vi "save config.vi"(8 "error in (no error)":errorcluster, 10 "file config":string, 11 "Channel in":refnum<class "Channel.lvclass">) -> (0 "error out":errorcluster, 3 "Channel out":refnum<class "Channel.lvclass">)   [LabVIEW 2018, in "Channel.lvclass"]
uses:
  Channel.lvclass
  Channel.lvclass/Channel.ctl
  <vilib>/Utility/config.llb/Write Key (String).vi
  Interface/Interface.lvclass
  <vilib>/Utility/config.llb/NI_LVConfig.lvlib
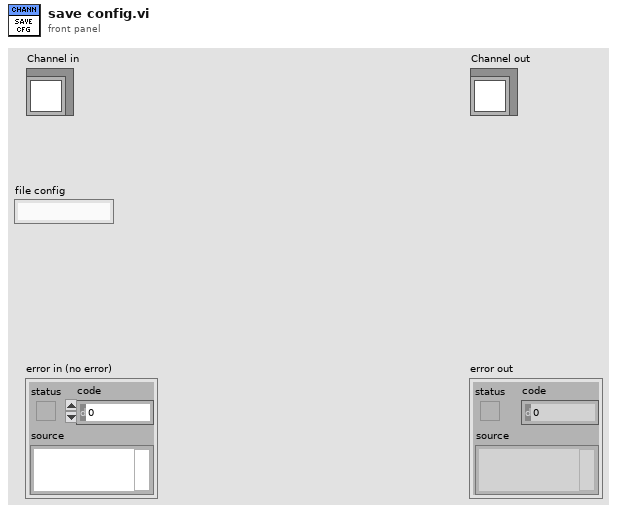
[diagram p1: front panel]
types:
  T1 = cluster{"ACQUISITION_MODE":u8, "TRIGGER_MODE":u8, "READ_MODE":u8, "PREAMP":u8, "READOUT_RATE":u8, "VERTICAL_SHIFT_SPEED":u8, "EM_MODE":u8, "EM_GAIN":u16, "SHUTTER_MODE":u8, "SHUTTER_TTL":u8, "SHUTTER_OPENNING_TIME":u16, "SHUTTER_CLOSING_TIME":u16, "VBIN":u16, "HBIN":u16, "INITIAL_LINE":u16, "INITIAL_COLUMN":u16, "FINAL_LINE":u16, "FINAL_COLUMN":u16, "FRAME_TRANSFER":bool, "VERTICAL_CLOCK_VOLTAGE":u8, "AD_CHANNEL":u32}
  T2 = typedef "NI_LVConfig.lvlib/Config Data RefNum.ctl" = refnum<k1>
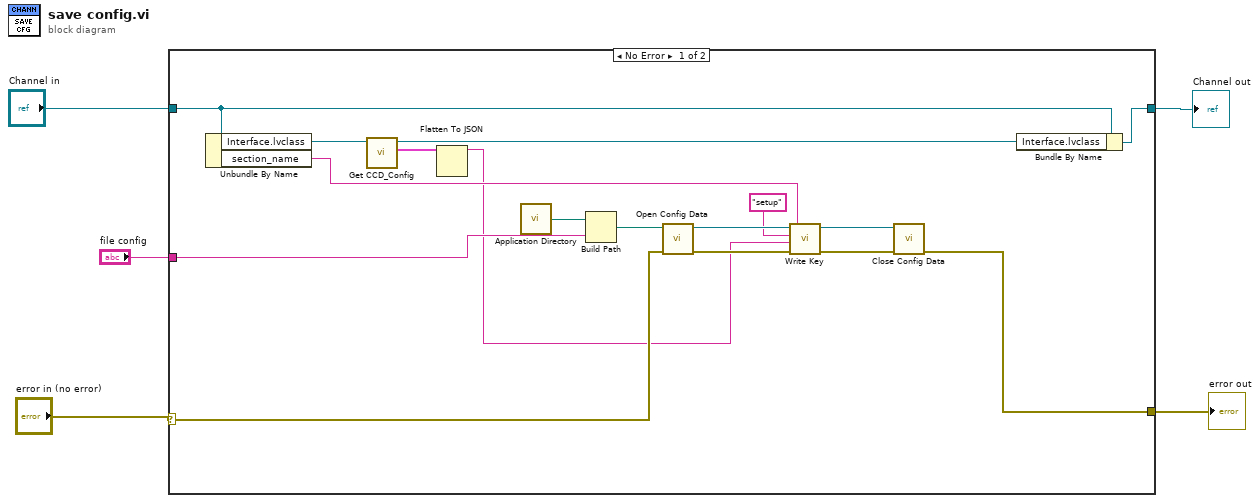
[diagram p0: block diagram]
diagram:
  n1 = case shown="No Error" "error in (no error)" {
    selector: "error in (no error)" -> [w15 w24]
    tunnel: [w7 w24] -> w2
    tunnel: [w16 w23] -> w3
    tunnel: "Channel in" -> [w17 w23]
    tunnel: "file config" -> [w10 _]
    frame No Error {
      n2 = Unbundle By Name(w17) -> ("Interface.lvclass"=w14:refnum<class "Interface.lvclass">, "section_name"=w20:string)
      n3 = call-dynamic "Get CCD_Config.vi"("Interface in"=w14) -> ("output cluster"=w9:T1, "Interface out"=w6:refnum<class "Interface.lvclass">)  [unwired: 8 in, 1 out]
      n4 = Flatten To JSON(anything=w9) -> (JSON string=w8:string)  [unwired: 2 in, 1 out]
      n5 = call <vilib>:"Application Directory.vi"() -> ("Application Directory"=w22:path)
      n6 = Build Path(base path=w22, name or relative path=w10) -> (appended path=w21:path)
      n7 = call <vilib>:"Open Config Data.vi"("error in (no error)"=w15, "configuration file path"=w21) -> ("error out"=w13:errorcluster, "refnum"=w19:T2)  [unwired: 7 in, 1 out]
      n8 = call-poly <vilib>:"Write Key.vi"("section"=w20, "error in (no error)"=w13, "value"=w8, "key"="setup", "refnum"=w19) -> ("error out"=w11:errorcluster, "refnum out"=w12:T2)  [unwired: 4 in, 1 out]
      n9 = call <vilib>:"Close Config Data.vi"("error in (no error)"=w11, "refnum"=w12) -> ("error out"=w7:errorcluster)  [unwired: 8 in, 1 out]
      n10 = Bundle By Name(cluster=w17, "Interface.lvclass"=w6) -> (w16:refnum<class "Channel.lvclass">)
    }
    frame Error {
    }
  }
  "error out" <- w2
  "Channel out" <- w3
